vi "Agilent 3352X Series Arbitrary Waveform Phase.vi"() -> ()   [LabVIEW 2019]
doc: "This example shows how to create then configure an phase of arbitrary waveform.\n\n<b>Note</b>:\nThis example is only available for 33600 series models."
uses:
  Instance           2 53Saved   Agilent 3352X Series Arbitrary Waveform Phase .vi
  Instance           1 53Saved   Agilent 3352X Series Arbitrary Waveform Phase .vi
  <instrlib>/Agilent 3352X Series/Agilent 3352X Series.lvlib
panel:
  in  "Sample Rate (40000 Sa/s)":dbl=40000.0
  in  "Phase Offset (0 Degree)":dbl
  in  "Units (0: Degree)":i32(ring) items=["Degree", "Radian", "Second", "Sample"]
  in  "Gain (0.1 Vpp)":dbl=0.1
  in  "Arbitrary Waveform Name":string="ARB1"
  in  "VISA resource name":refnum<visa-resource-name>
  # "(c) 2011-2021  National Instruments.  ALL RIGHTS RESERVED."
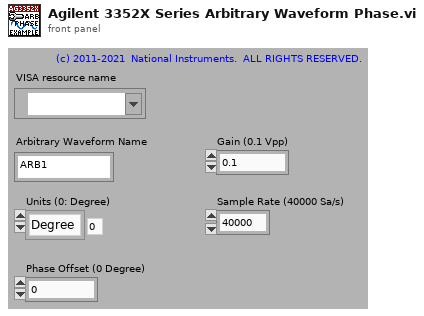
[diagram p1: front panel]
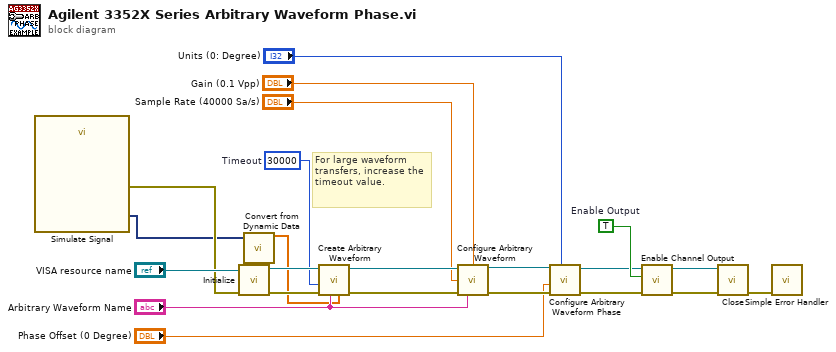
[diagram p0: block diagram]
diagram:
  w15 = TRUE  # Enable Output
  w10 = u32 30000  # Timeout
  # "For large waveform transfers, increase the timeout value."
  n1 = call "Simulate Signal"() -> ("Sine with Uniform Noise"=w2:dynamicdata, "error out"=w21:errorcluster)  [unwired: 8 in, 6 out]
  n2 = call <instrlib>:"Initialize.vi"("error in (no error)"=w21, "VISA resource name"="VISA resource name") -> ("error out"=w17:errorcluster, "VISA resource name out"=w16:refnum<visa-resource-name>)  [unwired: 2 in, 6 out]
  n3 = call "Convert from Dynamic Data"("Dynamic Data Type"=w2) -> ("Array"=w1:dbl[])  [unwired: 3 in]
  n4 = call <instrlib>:"Create Arbitrary Waveform.vi"("Arbitrary Waveform Data"=w1, "Arbitrary Waveform Name (ARB1)"="Arbitrary Waveform Name", "error in (no error)"=w17, "Timeout (10000 ms)"=w10, "VISA resource name"=w16) -> ("error out"=w13:errorcluster, "VISA resource name out"=w14:refnum<visa-resource-name>)  [unwired: 2 in, 3 out]
  n5 = call <instrlib>:"Configure Arbitrary Waveform.vi"("VISA resource name"=w14, "Amplitude (0.1 Vpp)"="Gain (0.1 Vpp)", "Sample Rate (40000 Sa/s)"="Sample Rate (40000 Sa/s)", "error in (no error)"=w13, "Arbitrary Waveform (ARB1)"="Arbitrary Waveform Name") -> ("VISA resource name out"=w9:refnum<visa-resource-name>, "error out"=w8:errorcluster)  [unwired: 5 in, 4 out]
  n6 = call <instrlib>:"Configure Arbitrary Waveform Phase.vi"("Units (0: Degree)"="Units (0: Degree)", "error in (no error)"=w8, "Phase Offset (0 Degree)"="Phase Offset (0 Degree)", "VISA resource name"=w9) -> ("error out"=w6:errorcluster, "VISA resource name out"=w7:refnum<visa-resource-name>)  [unwired: 1 in, 5 out]
  n7 = call <instrlib>:"Enable Channel Output.vi"("error in (no error)"=w6, "Enable Output (T: Enable)"=w15, "VISA resource name"=w7) -> ("error out"=w19:errorcluster, "VISA resource name out"=w18:refnum<visa-resource-name>)  [unwired: 2 in, 5 out]
  n8 = call <instrlib>:"Close.vi"("error in (no error)"=w19, "VISA resource name"=w18) -> ("error out"=w20:errorcluster)  [unwired: 9 out]
  n9 = call <vilib>:"Simple Error Handler.vi"("error in (no error)"=w20) -> ()  [unwired: 1 in, 8 out]
